vi "dsdll_output_play.vi"(8 "error in":errorcluster, 10 "looped mode (true)":bool=TRUE, 11 "dsdll instance in":T1={"dsdll path"=path "E:/LVprog/DirectSoundDLL/dsdll.dll", "dsdll handle"=[], "output devices"=[], "capture devices"=[]}) -> (0 "error out":errorcluster, 3 "dsdll instance out":T1)   [LabVIEW 2020, in "dsdll.lvlib"]
doc: "Call to start playback of previously loaded output device buffer (after using some of the 'dsdll_output_write...' VIs).\nThe 'looped mode' option enables playback of the waveform in an infinite loop. If set to false the waveform will be played just once. This VI can be called repeatedly."
uses:
  dsdll.lvlib
  dsdll_instance.ctl
  dsdll_device_record.ctl
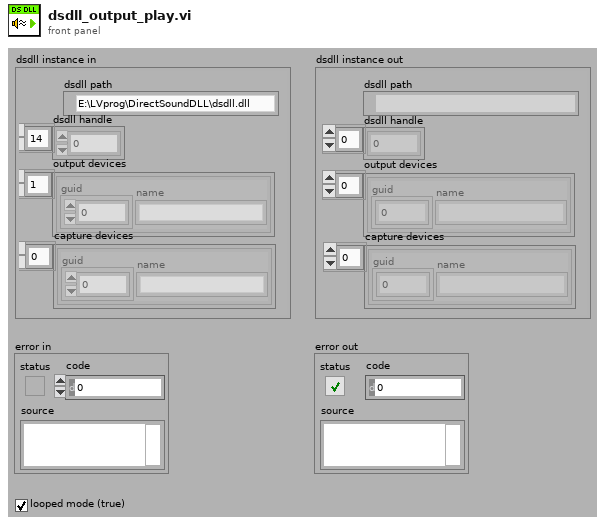
[diagram p1: front panel]
types:
  T1 = typedef "dsdll.lvlib/dsdll_instance.ctl" = cluster{"dsdll path":path, "dsdll handle":u8[], "output devices":T2[], "capture devices":T2[]}
  T2 = typedef "dsdll.lvlib/dsdll_device_record.ctl" = cluster{"guid":u8[], "name":string}
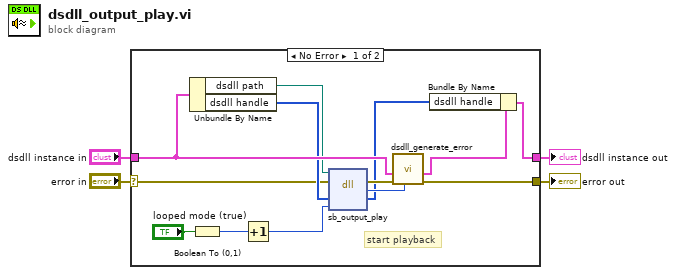
[diagram p0: block diagram]
diagram:
  n1 = case shown="No Error" "error in" {
    selector: "error in" -> [w8 w18]
    tunnel: "dsdll instance in" -> [w15 w19]
    tunnel: [w12 w18] -> w3
    tunnel: [w9 w19] -> w4
    frame No Error {
      # "start playback"
      n2 = Unbundle By Name(w15) -> ("dsdll path"=w14:path, "dsdll handle"=w13:u8[])
      n3 = Boolean To (0,1)(Boolean="looped mode (true)") -> (0, 1=w6:i16)
      n4 = Increment(x=w6) -> (x+1=w5:i16)
      n5 = dll-call lib="dsdll.dll" fn="sb_output_play" ("sb_get_handle_size()")(path in=w14, error in=w8, "handle"=w13, "mode"=w5) -> (error out=w17:errorcluster, "error"=w16:i32, "handle"=w10:u8[])  [unwired: 2 in, 1 out]
      n6 = call "dsdll_generate_error.vi"("error code"=w16, "error in"=w17, "dsdll instance in"=w15) -> ("error out"=w12:errorcluster, "dsdll instance out"=w11:T1)  [unwired: 6 in, 1 out]
      n7 = Bundle By Name(cluster=w11, "dsdll handle"=w10) -> (w9:T1)
    }
    frame Error {
    }
  }
  "error out" <- w3
  "dsdll instance out" <- w4
